vi "Zdrift.vi"() -> ()   [LabVIEW 2014]
doc: "This example records the Z channel (ie the tip height) and calculates the drift along this axis. The drift speed can then be applied to compensate for it.\nBefore starting the measurement, the tip must be in contact with the sample and the Z-Controller must be running.\n\n- Nanonis Programming Interface -"
uses:
  <userlib>/Nanonis Prog Interface V5/Nanonis Prog Interface.lvlib
panel:
  out "Drift":dbl
  in  "Duration":dbl=60.0 format="%.0g"
  # "Example program for the Nanonis programming interface\n\n-  Measure the drift speed along Z -"
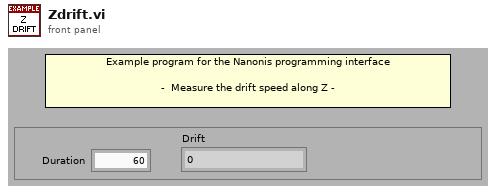
[diagram p1: front panel]
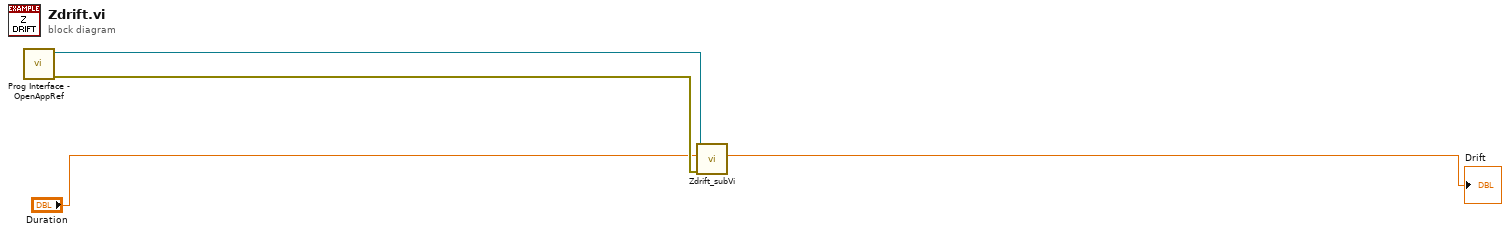
[diagram p0: block diagram]
diagram:
  n1 = call <userlib>:"Prog Interface - OpenAppRef.vi"() -> ("Error out"=w3:errorcluster, "Application reference"=w4:refnum<vi>)  [unwired: 6 in]
  n2 = call "Zdrift_subVi.vi"("error in (no error)"=w3, "Duration"="Duration", "Application in"=w4) -> ("z drift"=→"Drift":dbl)  [unwired: 6 in, 2 out]
